vi "Forcade_ZoomPictureShowSize.vi"(8 "error in (no error)":errorcluster caption="错误输入（无错误）", 10 "Bounds":T1, 11 "Picture_Class 输入":refnum<class "Picture_Class.lvclass"> caption="DNL_LabVIEW Object in") -> (0 "error out":errorcluster caption="错误输出", 1 "RealSize":T1, 2 "ZoomFactor":dbl, 3 "Picture_Class 输出":refnum<class "Picture_Class.lvclass"> caption="DNL_LabVIEW Object out")   [LabVIEW 2013, in "Picture_Class.lvclass"]
uses:
  Picture_Class.lvclass
  <vilib>/Utility/miscctls.llb/LVBoundsTypeDef.ctl
  Picture_Class.lvclass/Picture_Class.ctl
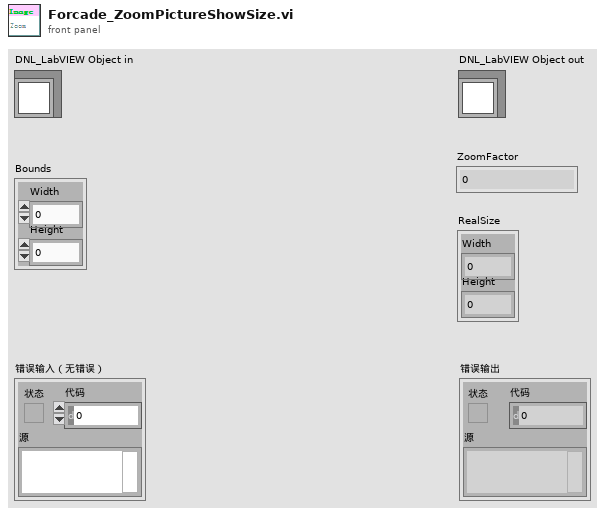
[diagram p1: front panel]
types:
  T1 = typedef "LVBoundsTypeDef.ctl" = cluster{"Width":u32, "Height":u32}
  T2 = typedef "imagedata.ctl" = cluster{"image type":i32, "image depth":i32, "image":u8[], "mask":u8[], "colors":u32[], "Rectangle":cluster{"left":i16, "top":i16, "right":i16, "bottom":i16}}
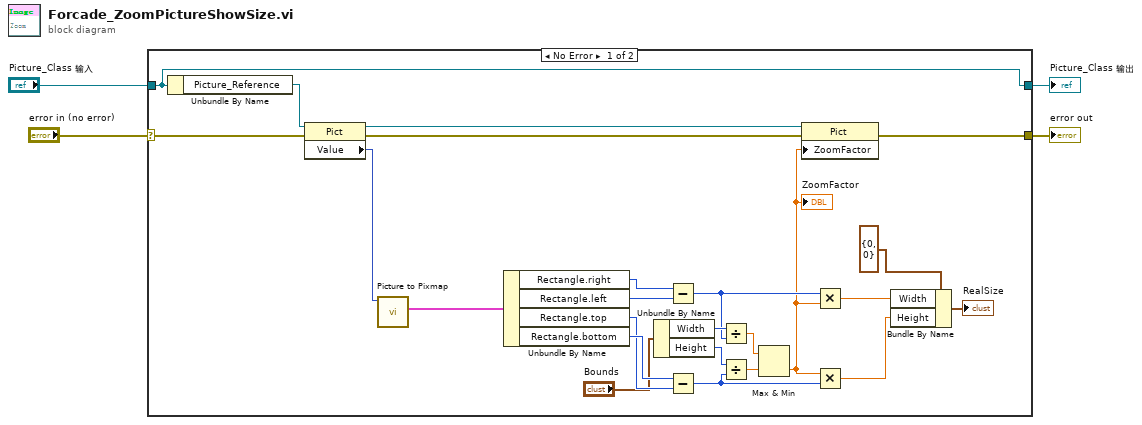
[diagram p0: block diagram]
diagram:
  n1 = case shown="No Error" "error in (no error)" {
    selector: "error in (no error)" -> [w26 w30]
    tunnel: [w13 w30] -> w3
    tunnel: [w28 w29] -> w1
    tunnel: "Picture_Class 输入" -> [w28 w29]
    frame No Error {
      n2 = Unbundle By Name(w28) -> ("Picture_Reference"=w27:refnum<vi>)
      n3 = property class="Pict"(reference=w27, error in=w26) -> (reference out=w15:refnum<vi>, error out=w14:errorcluster, "Value"=w25:picture)
      n4 = call <vilib>:"Picture to Pixmap.vi"("picture"=w25) -> ("image data"=w16:T2)  [unwired: 9 in, 1 out]
      n5 = Unbundle By Name(w16) -> ("Rectangle.right"=w17:i16, "Rectangle.left"=w18:i16, "Rectangle.top"=w19:i16, "Rectangle.bottom"=w20:i16)
      n6 = Unbundle By Name("Bounds") -> ("Width"=w21:u32, "Height"=w22:u32)
      n7 = Subtract(x=w17, y=w18) -> (x-y=w11:i16)
      n8 = Subtract(x=w20, y=w19) -> (x-y=w9:i16)
      n9 = Divide(x=w21, y=w11) -> (x/y=w24:dbl)
      n10 = Divide(x=w22, y=w9) -> (x/y=w23:dbl)
      n11 = Max & Min(x=w24, y=w23) -> (min(x,y)=w10:dbl)  [unwired: 1 out]
      "ZoomFactor" <- w10
      n12 = property class="Pict"(reference=w15, error in=w14, "ZoomFactor"=w10) -> (error out=w13:errorcluster)  [unwired: 1 out]
      n13 = Multiply(x=w11, y=w10) -> (x*y=w7:dbl)
      n14 = Multiply(x=w10, y=w9) -> (x*y=w5:dbl)
      n15 = Bundle By Name(cluster=T1 {"Width"=0, "Height"=0} ("RealSize 2"), "Width"=w7, "Height"=w5) -> (→"RealSize":T1)
    }
    frame Error {
    }
  }
  "error out" <- w3
  "Picture_Class 输出" <- w1
